vi "MSEncoder SubVI Q2Beta.vi"(10 "q_z":dbl) -> (2 "Beta":dbl)   [LabVIEW 2018]
uses:
  <vilib>/Analysis/NI_AALPro.lvlib
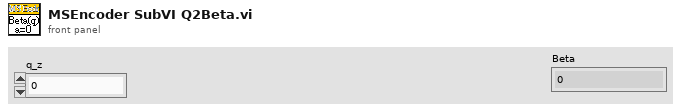
[diagram p1: front panel]
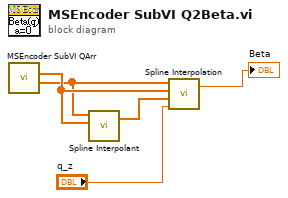
[diagram p0: block diagram]
diagram:
  n1 = call "MSEncoder SubVI QArr.vi"() -> ("Beta"=w1:dbl[], "Q"=w4:dbl[])  [unwired: 10 in]
  n2 = call <vilib>:"Spline Interpolant.vi"("X"=w4, "Y"=w1) -> ("Interpolant"=w5:dbl[])  [unwired: 2 in, 1 out]
  n3 = call <vilib>:"Spline Interpolation.vi"("x value"="q_z", "Interpolant"=w5, "X"=w4, "Y"=w1) -> ("interpolation value"=→"Beta":dbl)  [unwired: 1 out]
